vi "UDP-Custom-Device.Async.vi"(10 "Parameters":variant, 11 "Process":refnum<class "Process.lvclass">) -> ()   [LabVIEW 2015, in "UDP-Custom-Device Engine.lvlib"]
uses:
  UDP-Custom-Device Engine.lvlib
  <vilib>/NI/NIVS Inline Async API/_VS Inline Async API/Process/Process.lvclass
  <vilib>/NI/NIVS Inline Async API/_VS Inline Async API/Process/Process.lvclass/Process.ctl
  <vilib>/NI/NIVS Inline Async API/_Data Access Engine/Access Type Classes/Read/Read.lvclass/Read.ctl
  <vilib>/NI/NIVS Inline Async API/_Data Access Engine/Access Type Classes/Write/Write.lvclass/Write.ctl
  <vilib>/NI/NIVS Inline Async API/_Data Access Engine/Data Access Engine/Methods/Write.Data.vi
  <vilib>/NI/NIVS Inline Async API/_Data Access Engine/Data Access Engine/Methods/Read.Data.vi
  <vilib>/NI/NIVS Inline Async API/_VS Inline Async API/Error Handling Process/SubVIs/Error.ConvertArray.vi
  <vilib>/NI/NIVS Inline Async API/_Data Access Engine/Access Type Classes/Write/Write.ProcessData.vi
  <vilib>/NI/NIVS Inline Async API/_Data Access Engine/Access Type Classes/Read/Read.ProcessData.vi
  <vilib>/NI/NIVS Inline Async API/_Data Access Engine/Data Access Engine/Data Access Engine.lvclass
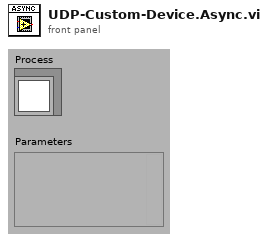
[diagram p1: front panel]
types:
  T1 = typedef "UDP-Custom-Device Engine.lvlib/RTStateVariables.ctl" = cluster{"Async":refnum<class "VS Inline Async API.lvclass">, "Settings":T2, "Connection ID":refnum<k16>, "Rx FIFO Ref":T5, "Tx FIFO Ref":T6}
  T2 = typedef "UDP-Custom-Device Shared.lvlib/Compiled.Settings.ctl" = cluster{"Name":string, "Rx FIFO Polling Rate":u32, "Rx FIFO Timeout":u32, "Destination Address":string, "Local Address":string, "Server Port":u16, "Tx Enabled?":bool, "Rx Enabled?":bool, "Rx Packet Info":T3[], "Tx Packet Info":T4[]}
  T3 = typedef "UDP-Custom-Device Shared.lvlib/Rx.PacketInfo.ctl" = cluster{"Packet Name":string, "Packet ID":i32, "Timeout":i32, "Rx IP Address":string, "Rx Port":i32}
  T4 = typedef "UDP-Custom-Device Shared.lvlib/Tx.PacketInfo.ctl" = cluster{"Packet Name":string, "Packet ID":i32, "Decimation":i32, "Destination IP Address":string, "Destination Port":i32}
  T5 = typedef "Data Access Engine.lvlib/Data Access Engine.lvclass/Write.DVR.ctl" = refnum<data-value>
  T6 = typedef "Data Access Engine.lvlib/Data Access Engine.lvclass/Read.DVR.ctl" = refnum<data-value>
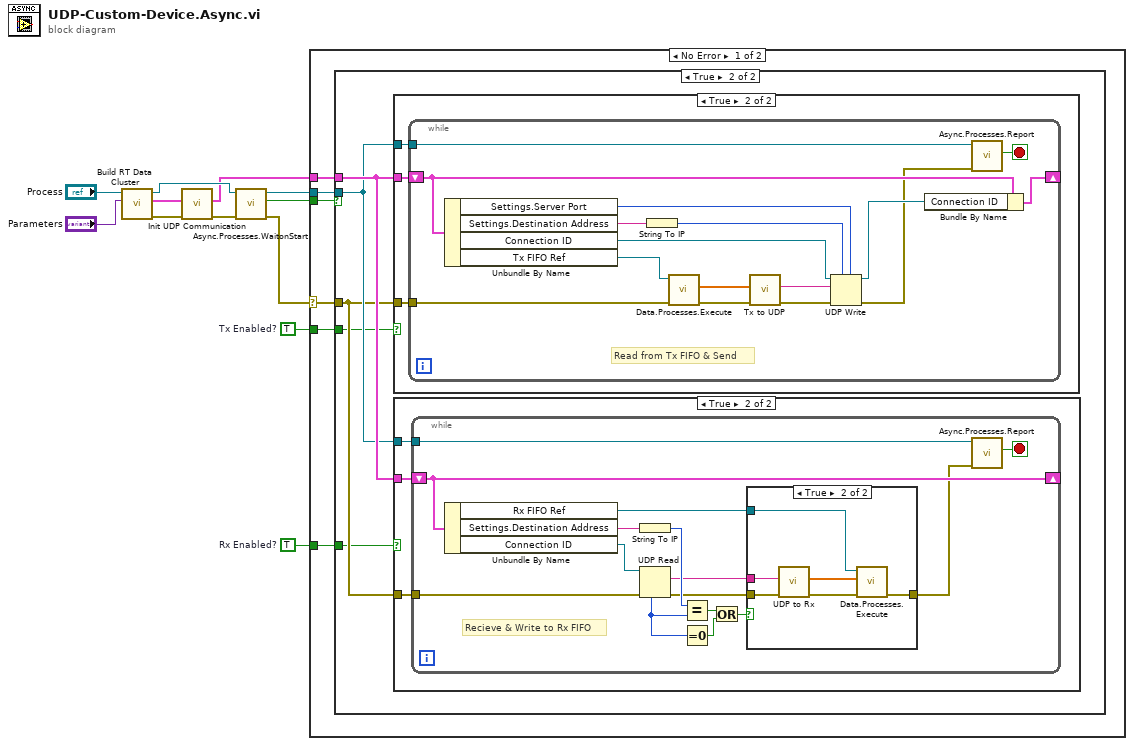
[diagram p0: block diagram]
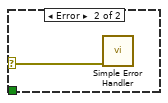
[diagram p6: hidden frame]
diagram:
  w1 = TRUE  # Tx Enabled?
  w2 = TRUE  # Rx Enabled?
  n1 = call "Build RT Data Cluster.vi"("Compiled Settings Parameters"="Parameters", "Process In"="Process") -> ("error out"=w7:errorcluster, "RT State Variables"=w5:T1, "Process Out"=w6:refnum<class "Process.lvclass">)  [unwired: 7 in]
  n2 = call "Init UDP Communication.vi"("error in (no error)"=w7, "RT State Variables In"=w5) -> ("error out"=w4:errorcluster, "RT State Variables Out"=w3:T1)  [unwired: 8 in]
  n3 = call <vilib>:"Async.Processes.WaitonStart.vi"("error in (no error)"=w4, "Process"=w6) -> ("error out"=w10:errorcluster, "Execute"=w12:bool, "Process out"=w11:refnum<class "Process.lvclass">)  [unwired: 7 in]
  n4 = case shown="No Error" w10 {
    selector: w10 -> [w16 w68]
    tunnel: w12 -> [w18 _]
    tunnel: w11 -> [w17 _]
    tunnel: w3 -> [w15 _]
    tunnel: w2 -> [w14 _]
    tunnel: w1 -> [w13 _]
    frame No Error {
      n5 = case shown="True" w18 {
        tunnel: w16 -> [_ w21]
        tunnel: w17 -> [_ w22]
        tunnel: w15 -> [_ w23]
        tunnel: w14 -> [_ w20]
        tunnel: w13 -> [_ w19]
        frame False {
        }
        frame True {
          n6 = case shown="True" w19 {
            tunnel: w23 -> [_ w26]
            tunnel: w22 -> [_ w25]
            tunnel: w21 -> [_ w24]
            frame False {
            }
            frame True {
              n7 = while {
                tunnel: w24 -> [w39]
                tunnel: w25 -> [w42]
                shift-right: [w29] -> _
                shift-left: w26 -> [w30]
                stop <- w41 stop-if-true
                # "Read from Tx FIFO & Send"
                n8 = Unbundle By Name(w30) -> ("Settings.Server Port"=w31:u16, "Settings.Destination Address"=w34:string, "Connection ID"=w33:refnum<k16>, "Tx FIFO Ref"=w40:T6)
                n9 = String To IP(1:w34) -> (0:w32:u32)
                n10 = call-poly <vilib>:"Data.Processes.Execute.vi"("error in (no error)"=w39, "Ref"=w40) -> ("error out"=w38:errorcluster, "Values"=w37:dbl[])  [unwired: 7 in, 1 out]
                n11 = call "Tx to UDP.vi"("error in (no error)"=w38, "Tx Array"=w37) -> ("error out"=w36:errorcluster, "Tx String"=w35:string)  [unwired: 8 in]
                n12 = UDP Write(address=w32, port or service name=w31, connection ID=w33, data in=w35, 8:w36) -> (error out=w27:errorcluster, 3:w28:refnum<k16>)  [unwired: 1 in]
                n13 = Bundle By Name(cluster=w30, "Connection ID"=w28) -> (w29:T1)
                n14 = call <vilib>:"Async.Processes.Report.vi"("Error"=w27, "Process in"=w42) -> ("Stop"=w41:bool)  [unwired: 8 in, 1 out]
              }
            }
          }
          n15 = case shown="True" w20 {
            tunnel: w23 -> [_ w45]
            tunnel: w22 -> [_ w44]
            tunnel: w21 -> [_ w43]
            frame False {
            }
            frame True {
              n16 = while {
                tunnel: w43 -> [w57]
                tunnel: w44 -> [w60]
                shift-right: [w58] -> _
                shift-left: w45 -> [w58]
                stop <- w59 stop-if-true
                # "Recieve & Write to Rx FIFO"
                n17 = Unbundle By Name(w58) -> ("Rx FIFO Ref"=w48:T5, "Settings.Destination Address"=w55:string, "Connection ID"=w56:refnum<k16>)
                n18 = String To IP(1:w55) -> (0:w54:u32)
                n19 = UDP Read(connection ID=w56, 8:w57) -> (data out=w47:string, error out=w49:errorcluster, 6:w53:u32)  [unwired: 2 in, 2 out]
                n20 = Equal?(x=w54, y=w53) -> (x = y?=w52:bool)
                n21 = Equal To 0?(x=w53) -> (x = 0?=w51:bool)
                n22 = Or(x=w52, y=w51) -> (x .or. y?=w50:bool)
                n23 = case shown="True" w50 {
                  tunnel: w49 -> [w61 w65]
                  tunnel: [w61 w66] -> w46
                  tunnel: w48 -> [_ w67]
                  tunnel: w47 -> [_ w62]
                  frame False {
                  }
                  frame True {
                    n24 = call "UDP to Rx.vi"("error in (no error)"=w65, "Rx String"=w62) -> ("error out"=w64:errorcluster, "Rx Array"=w63:dbl[])  [unwired: 8 in]
                    n25 = call-poly <vilib>:"Data.Processes.Execute.vi"("error in (no error)"=w64, "Values"=w63, "Ref"=w67) -> ("error out"=w66:errorcluster)  [unwired: 8 in]
                  }
                }
                n26 = call <vilib>:"Async.Processes.Report.vi"("Error"=w46, "Process in"=w60) -> ("Stop"=w59:bool)  [unwired: 8 in, 1 out]
              }
            }
          }
        }
      }
    }
    frame Error {
      n27 = call <vilib>:"Simple Error Handler.vi"("error in (no error)"=w68) -> ()  [unwired: 4 in, 5 out]
    }
  }
